vi "MB Ethernet Example Master (Legacy).vi"() -> ()   [LabVIEW 2023, in "Voegtlin_NI_SMART_Modbus_Drivers.lvlib"]
uses:
  Voegtlin_NI_SMART_Modbus_Drivers.lvlib
  MB Modbus Command.ctl
panel:
  in  "Remote Port":u16=502
  in  "Remote IP Address":string="127.0.0.1"
  in  "Stop":bool
  out "Slave Input Registers":u16[](array[numeric]) caption="Slave Input Registers (Read Only)"
  out "Slave Discrete Inputs":bool[](array[boolean])
  in  "Coils to Write":bool[](array[boolean])=[FALSE, FALSE, FALSE, FALSE]
  in  "Registers to Write":u16[](array[numeric])=[0, 0, 0, 0]
  # "MB Ethernet Example Master.vi\n\nInstructions\n1. Run MB Ethernet Example Slave.vi\n2. Run this VI.\n3. Modify the discrete inputs or input registers on the slave -> they're updated on the master.\n4. Modify the coils and registers on the master -> they're updated on the slave."
  # "Data to write to the slave"
  # "Slave Read-only Registers"
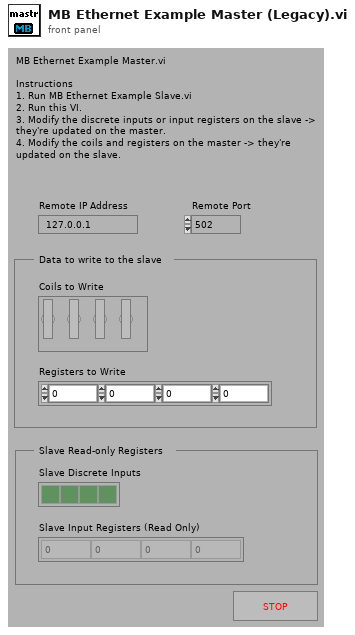
[diagram p1: front panel]
types:
  T1 = typedef "Voegtlin_NI_SMART_Modbus_Drivers.lvlib/MB Modbus Command.ctl" = cluster{"Function Code":u8, "Starting Address":u16, "Quantity":u16, "Data":u16[], "Discrete":bool[]}
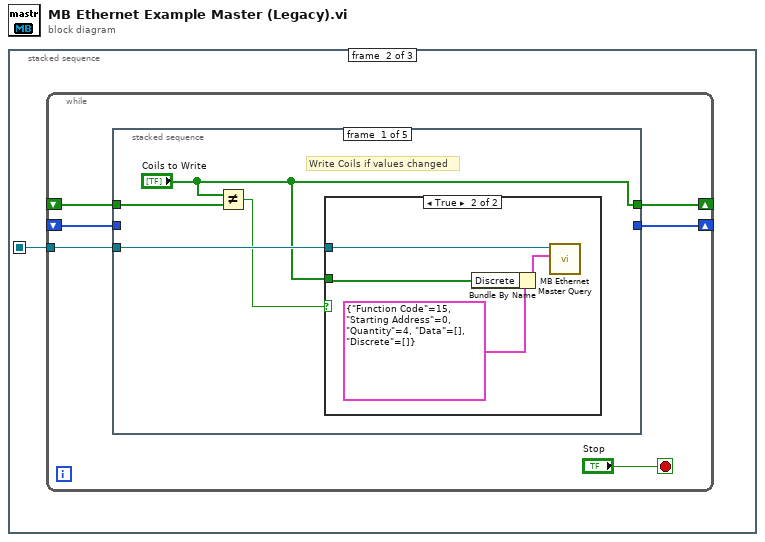
[diagram p0: block diagram]
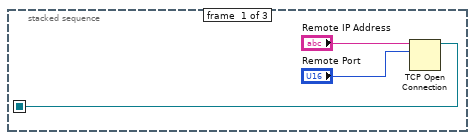
[diagram p2: hidden frame]
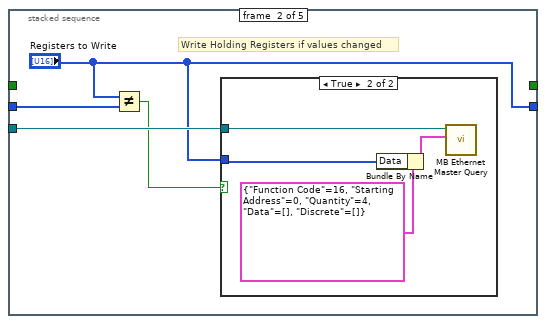
[diagram p4: hidden frame]
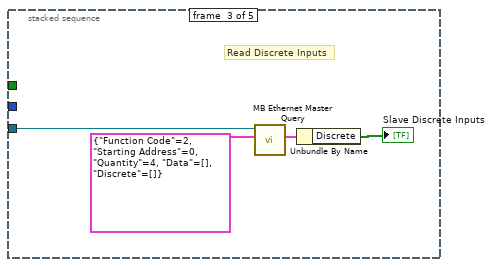
[diagram p6: hidden frame]
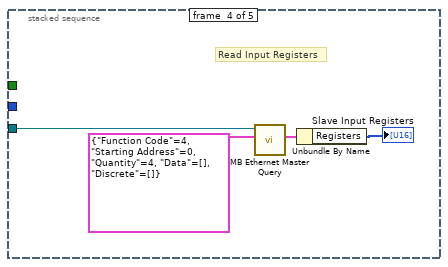
[diagram p7: hidden frame]
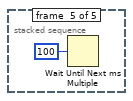
[diagram p8: hidden frame]
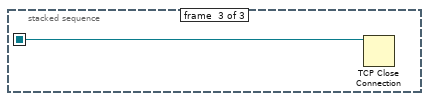
[diagram p9: hidden frame]
diagram:
  n1 = stacked-sequence {
    seq-local: [w1 _ _] -> [_ w4 w36]
    frame #0 {
      n2 = TCP Open Connection(address="Remote IP Address", remote port or service name="Remote Port") -> (connection ID=w1:refnum<k5>)  [unwired: 1 in, 3 out]
    }
    frame #1 {
      n3 = while {
        tunnel: w4 -> [w10]
        shift-right: [w8] -> _
        shift-left: _ -> [w9]
        shift-right: [w6] -> _
        shift-left: _ -> [w7]
        stop <- "Stop" stop-if-true
        n4 = stacked-sequence {
          tunnel: w10 -> [w14 w22 w30 w34 _]
          tunnel: w9 -> [w13 _ _ _ _]
          tunnel: ["Coils to Write" _ _ _ _] -> w8
          tunnel: w7 -> [_ w20 _ _ _]
          tunnel: [_ "Registers to Write" _ _ _] -> w6
          frame #0 {
            # "Write Coils if values changed"
            n5 = Not Equal?(x="Coils to Write", y=w13) -> (x != y?=w11:bool)
            n6 = case shown="True" w11 {
              tunnel: w14 -> [_ w16]
              tunnel: "Coils to Write" -> [_ w15]
              frame False {
              }
              frame True {
                n7 = Bundle By Name(cluster=T1 {"Function Code"=15, "Starting Address"=0, "Quantity"=4, "Data"=[], "Discrete"=[]} ("MODBUS Command"), "Discrete"=w15) -> (w17:T1)
                n8 = call "MB Ethernet Master Query.vi"("Modbus Command"=w17, "TCP Connection Refnum in"=w16) -> ()  [unwired: 5 in, 5 out]
              }
            }
          }
          frame #1 {
            # "Write Holding Registers if values changed"
            n9 = Not Equal?(x="Registers to Write", y=w20) -> (x != y?=w21:bool)
            n10 = case shown="True" w21 {
              tunnel: w22 -> [_ w24]
              tunnel: "Registers to Write" -> [_ w23]
              frame False {
              }
              frame True {
                n11 = Bundle By Name(cluster=T1 {"Function Code"=16, "Starting Address"=0, "Quantity"=4, "Data"=[], "Discrete"=[]} ("MODBUS Command"), "Data"=w23) -> (w25:T1)
                n12 = call "MB Ethernet Master Query.vi"("Modbus Command"=w25, "TCP Connection Refnum in"=w24) -> ()  [unwired: 5 in, 5 out]
              }
            }
          }
          frame #2 {
            # "Read Discrete Inputs"
            n13 = call "MB Ethernet Master Query.vi"("Modbus Command"=T1 {"Function Code"=2, "Starting Address"=0, "Quantity"=4, "Data"=[], "Discrete"=[]} ("MODBUS Command"), "TCP Connection Refnum in"=w30) -> ("Registers"=w29:cluster{"Registers":u16[], "Discrete":bool[]})  [unwired: 5 in, 4 out]
            n14 = Unbundle By Name(w29) -> ("Discrete"=→"Slave Discrete Inputs":bool[])
          }
          frame #3 {
            # "Read Input Registers"
            n15 = call "MB Ethernet Master Query.vi"("Modbus Command"=T1 {"Function Code"=4, "Starting Address"=0, "Quantity"=4, "Data"=[], "Discrete"=[]} ("MODBUS Command"), "TCP Connection Refnum in"=w34) -> ("Registers"=w33:cluster{"Registers":u16[], "Discrete":bool[]})  [unwired: 5 in, 4 out]
            n16 = Unbundle By Name(w33) -> ("Registers"=→"Slave Input Registers":u16[])
          }
          frame #4 {
            n17 = Wait Until Next ms Multiple(millisecond multiple=u32 100) -> ()  [unwired: 1 out]
          }
        }
      }
    }
    frame #2 {
      n18 = TCP Close Connection(connection ID=w36) -> ()  [unwired: 1 in, 3 out]
    }
  }
